vi "ScopeIntegrateSignal_v3.vi"() -> ()   [LabVIEW 2018]
doc: "This example illustrates how to use autosetup and continuously acquires waveforms from a single channel using the following steps:\n\n1. Specify a valid VISA session. \n2. Specify a channel. \n3. Specify a time-out value for reading waveform.\n4. Run the VI. The graph displays the waveform you acquire."
uses:
  <vilib>/Analysis/baseanly.llb/Mean (DBL).vi
  <instrlib>/Tektronix DPO MSO 2000 4000 Series/Public/Data/Read (Single Waveform).vi
  <vilib>/Waveform/WDTFileIO.llb/Export Waveform To Spreadsheet File.vi
  <instrlib>/Tektronix DPO MSO 2000 4000 Series/Tektronix DPO MSO 2000 4000 Series.lvlib
  <vilib>/Analysis/NI_AALBase.lvlib
panel:
  in  "Save waveform?":bool
  in  "autocurs":bool=TRUE
  out "roi_stop":i64=496919
  out "roi_start":i64=496793
  in  "thresh":dbl=0.30000000000000004 format="%#_13g"
  in  "acquire":bool=TRUE
  in  "milliseconds to wait":u32=100
  out "Numeric":i32
  out "standard deviation":dbl=-0.0 format="%0.2f"
  out "mean":dbl=nan format="%0.2f"
  in  "Looping?":bool
  in  "stop":bool
  out "integrated signal array":dbl[](array[numeric])=[5.081550747205201e-09]
  out "bkgd":dbl=-0.0005882788252936317 format="%0.5f"
  out "bkgd stop":dbl=0.00019852
  out "bkgd start":dbl=5.636363636363637e-05
  out "dt":dbl=4e-10
  out "integral (nVs)":sgl=5.0815506
  out "stop int":dbl=0.00019876854
  out "start int":dbl=0.00019871893000000001
  in  "Channel (0: Channel 1)":u16(ring)=2 items=["Channel 1", "Channel 2", "Channel 3", "Channel 4", "Math", "Reference 1", "Reference 2", "Reference 3", "Reference 4"]
  in  "Maximum Time (10000ms)":u32=10000
  in  "VISA Resource Name":refnum<visa-resource-name>="mdo4034c"
  out "Waveform Graph":waveform(dbl)(graph)={"t0"=timestamp(-0.0001988000000000545 s since 1904-01-01), "dt"=4e-10, "Y"=array[1000000 elements]}
  # "(C) 2006 - 2022. National Instruments Corporation. ALL RIGHTS RESERVED."
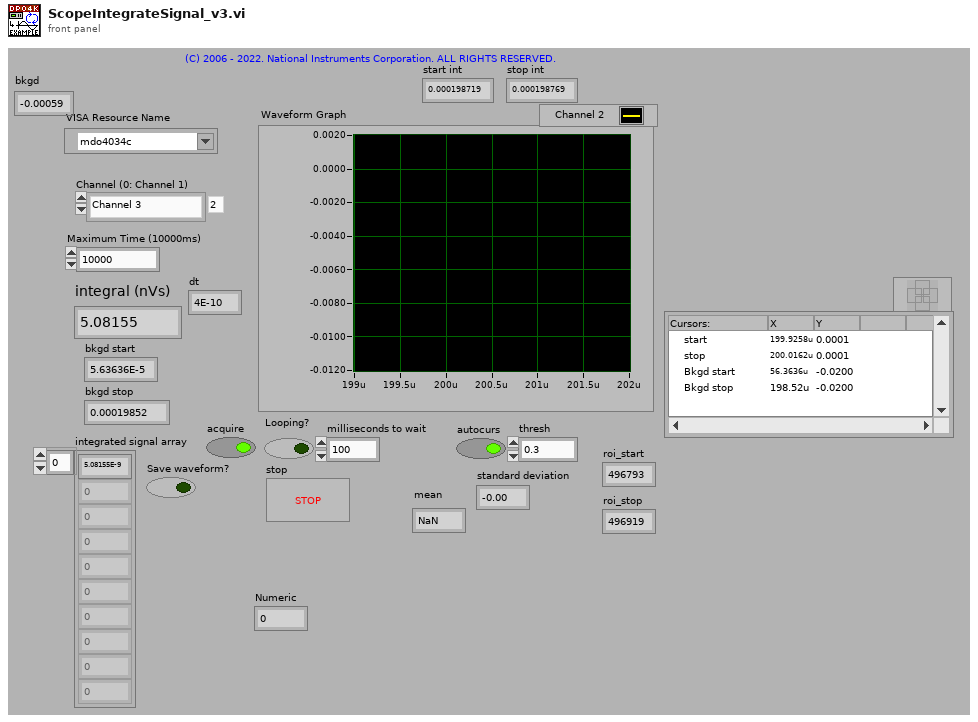
[diagram p1: front panel]
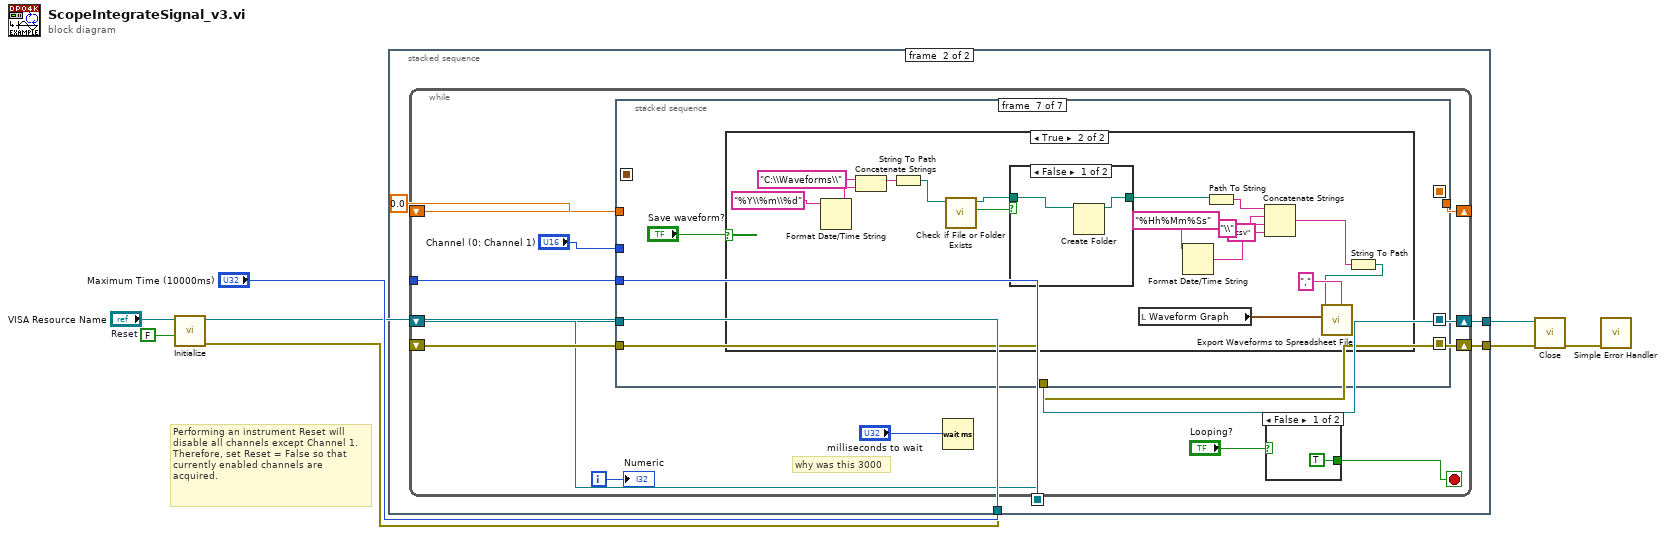
[diagram p0: block diagram]
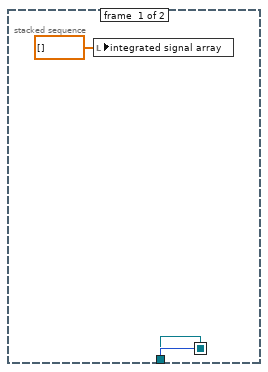
[diagram p2: hidden frame]
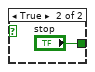
[diagram p3: hidden frame]
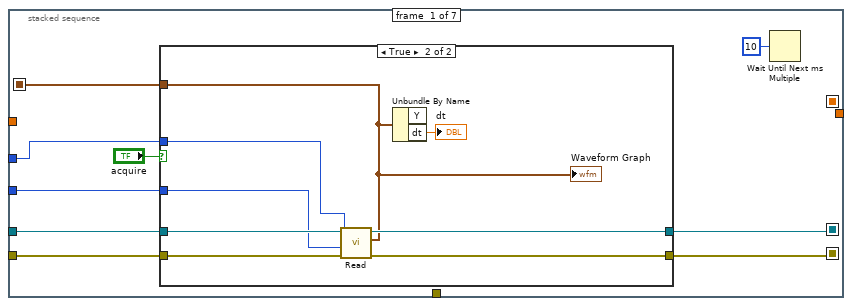
[diagram p4: hidden frame]
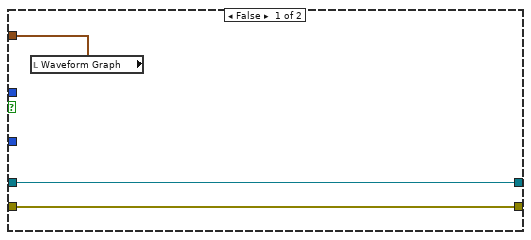
[diagram p5: hidden frame]
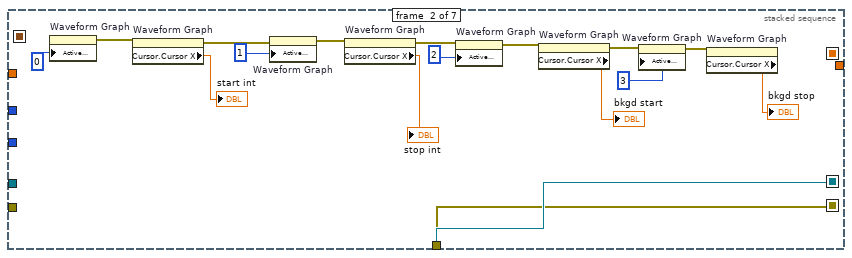
[diagram p6: hidden frame]
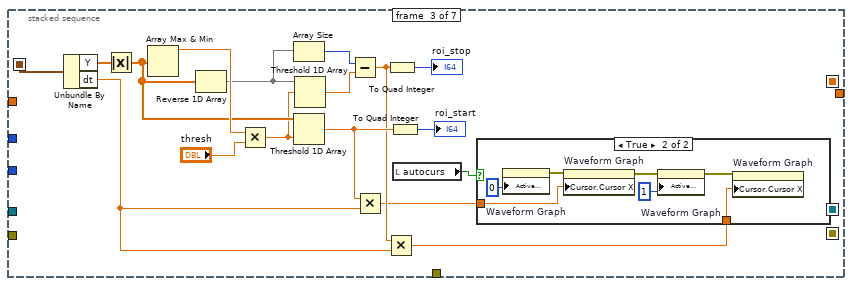
[diagram p7: hidden frame]
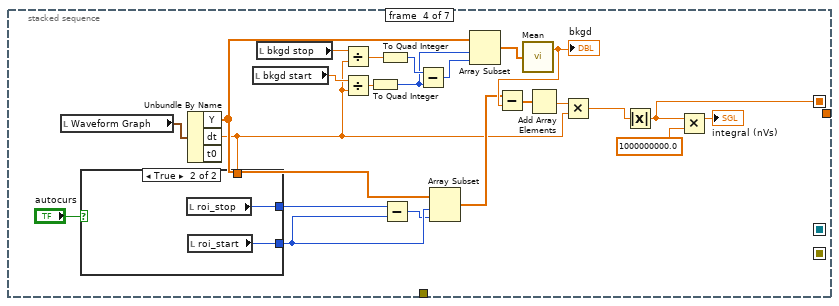
[diagram p9: hidden frame]
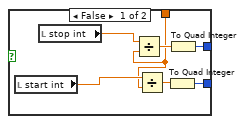
[diagram p10: hidden frame]
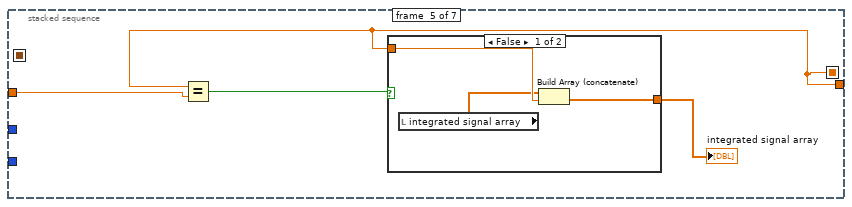
[diagram p11: hidden frame]
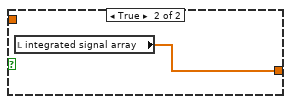
[diagram p12: hidden frame]
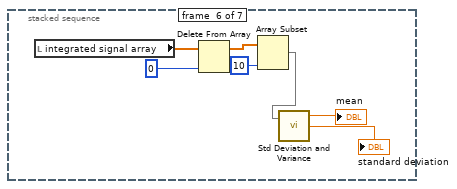
[diagram p13: hidden frame]
diagram:
  w4 = FALSE  # Reset
  # "Performing an instrument Reset will disable all channels except Channel 1. Therefore, set Reset = False so that currently enabled channels are acquired."
  n1 = call <instrlib>:"Initialize.vi"("Reset (True)"=w4, "VISA resource name"="VISA Resource Name") -> ("error out"=w2:errorcluster, "VISA resource name out"=w1:refnum<visa-resource-name>)  [unwired: 8 in]
  n2 = stacked-sequence {
    seq-local: [w12 _] -> [_ w16]
    seq-local: [w11 _] -> [_ w15]
    seq-local: [w10 _] -> [_ w14]
    tunnel: "Maximum Time (10000ms)" -> [w12 _]
    tunnel: w2 -> [w11 _]
    tunnel: w1 -> [w10 _]
    tunnel: [_ w18] -> w7
    tunnel: [_ w17] -> w6
    frame #0 {
      n3 = local write "integrated signal array"(dbl[] [] ("integrated signal array")) -> ()
    }
    frame #1 {
      n4 = while {
        tunnel: w16 -> [w28]
        shift-right: [w29] -> w17
        shift-left: w15 -> [w27]
        shift-right: [w30] -> w18
        shift-left: w14 -> [w26]
        shift-right: [w25] -> _
        shift-left: 0.0 -> [w24]
        i -> [w21]
        stop <- w22 stop-if-true
        # "why was this 3000"
        n5 = stacked-sequence {
          seq-local: [w39 _ _ _ _ _ _] -> [_ w69 _ _ _ _ _]
          seq-local: [w37 _ _ _ _ _ _] -> [_ w68 _ _ _ _ _]
          seq-local: [_ _ _ w101 _ _ _] -> [_ _ _ _ w127 _ _]
          seq-local: [w33 _ _ _ _ _ _] -> [_ _ w86 _ _ _ _]
          tunnel: w26 -> [w41 _ _ _ _ _ _]
          tunnel: w27 -> [w40 _ _ _ _ _ _]
          tunnel: w28 -> [w36 _ _ _ _ _ _]
          tunnel: "Channel (0: Channel 1)" -> [w35 _ _ _ _ _ _]
          tunnel: [_ w69 _ _ _ _ _] -> w30
          tunnel: [_ w68 _ _ _ _ _] -> w29
          tunnel: [_ _ _ _ w127 _ _] -> w25
          tunnel: w24 -> [_ _ _ _ w126 _ _]
          frame #0 {
            n6 = case shown="True" "acquire" {
              tunnel: w41 -> [w44 w52]
              tunnel: w40 -> [w43 w51]
              tunnel: [w44 w50] -> w39
              tunnel: [w43 w49] -> w37
              tunnel: w36 -> [_ w48]
              tunnel: w35 -> [_ w46]
              tunnel: [w42 w45] -> w33
              frame False {
                n7 = local read "Waveform Graph"() -> (w42:waveform(dbl))
              }
              frame True {
                n8 = call-poly <instrlib>:"Read.vi"("error in (no error)"=w51, "Maximum Time (10000ms)"=w48, "Channel (0: Channel 1)"=w46, "VISA resource name"=w52) -> ("error out"=w49:errorcluster, "Waveform Graph"=w45:waveform(dbl), "VISA resource name out"=w50:refnum<visa-resource-name>)  [unwired: 5 in]
                "Waveform Graph" <- w45
                n9 = Unbundle By Name(w45) -> ("dt"=→"dt":dbl)  [unwired: 1 out]
              }
            }
            n10 = Wait Until Next ms Multiple(millisecond multiple=u32 10) -> ()  [unwired: 1 out]
          }
          frame #1 {
            n11 = property on="Waveform Graph" class="WFGraph (strict)"("Active Cursor"=0 ("Cursor.Cursor Index")) -> (error out=w66:errorcluster)  [unwired: 2 in, 1 out]
            n12 = property on="Waveform Graph" class="WFGraph (strict)"(error in=w66) -> (error out=w65:errorcluster, "Cursor.Cursor X"=→"start int":dbl)  [unwired: 1 in, 1 out]
            n13 = property on="Waveform Graph" class="WFGraph (strict)"(error in=w65, "Active Cursor"=1 ("Cursor.Cursor Index")) -> (error out=w64:errorcluster)  [unwired: 1 in, 1 out]
            n14 = property on="Waveform Graph" class="WFGraph (strict)"(error in=w64) -> (error out=w59:errorcluster, "Cursor.Cursor X"=→"stop int":dbl)  [unwired: 1 in, 1 out]
            n15 = property on="Waveform Graph" class="WFGraph (strict)"(error in=w59, "Active Cursor"=u32 2) -> (error out=w60:errorcluster)  [unwired: 1 in, 1 out]
            n16 = property on="Waveform Graph" class="WFGraph (strict)"(error in=w60) -> (error out=w56:errorcluster, "Cursor.Cursor X"=→"bkgd start":dbl)  [unwired: 1 in, 1 out]
            n17 = property on="Waveform Graph" class="WFGraph (strict)"(error in=w56, "Active Cursor"=u32 3) -> (error out=w57:errorcluster)  [unwired: 1 in, 1 out]
            n18 = property on="Waveform Graph" class="WFGraph (strict)"(error in=w57) -> ("Cursor.Cursor X"=→"bkgd stop":dbl)  [unwired: 1 in, 2 out]
          }
          frame #2 {
            n19 = Unbundle By Name(w86) -> ("Y"=w85:dbl[], "dt"=w73:dbl)
            n20 = Absolute Value(x=w85) -> (abs(x)=w82:dbl[])
            n21 = Array Max & Min(array=w82) -> (max value=w84:dbl)  [unwired: 3 out]
            n22 = Reverse 1D Array(array=w82) -> (reversed array=w80:dbl[])
            n23 = Multiply(x=w84, y="thresh") -> (x*y=w81:dbl)
            n24 = Array Size(array=w80) -> (size(s)=w79:i32)
            n25 = Threshold 1D Array(2:w81, 3:w82) -> (0:w75:dbl)  [unwired: 1 in]
            n26 = Threshold 1D Array(2:w81, 3:w80) -> (0:w78:dbl)  [unwired: 1 in]
            n27 = Subtract(x=w79, y=w78) -> (x-y=w74:dbl)
            n28 = Multiply(x=w75, y=w73) -> (x*y=w71:dbl)
            n29 = Multiply(x=w74, y=w73) -> (x*y=w72:dbl)
            n30 = To Quad Integer(1:w74) -> (0:→"roi_stop":i64)
            n31 = To Quad Integer(1:w75) -> (0:→"roi_start":i64)
            n32 = local read "autocurs"() -> (w70:bool)
            n33 = case shown="True" w70 {
              tunnel: w72 -> [_ w88]
              tunnel: w71 -> [_ w87]
              frame False {
              }
              frame True {
                n34 = property on="Waveform Graph" class="WFGraph (strict)"("Active Cursor"=0 ("Cursor.Cursor Index")) -> (error out=w93:errorcluster)  [unwired: 2 in, 1 out]
                n35 = property on="Waveform Graph" class="WFGraph (strict)"(error in=w93, "Cursor.Cursor X"=w87) -> (error out=w92:errorcluster)  [unwired: 1 in, 1 out]
                n36 = property on="Waveform Graph" class="WFGraph (strict)"(error in=w92, "Active Cursor"=1 ("Cursor.Cursor Index")) -> (error out=w91:errorcluster)  [unwired: 1 in, 1 out]
                n37 = property on="Waveform Graph" class="WFGraph (strict)"(error in=w91, "Cursor.Cursor X"=w88) -> ()  [unwired: 1 in, 2 out]
              }
            }
          }
          frame #3 {
            n38 = local read "Waveform Graph"() -> (w113:waveform(dbl))
            n39 = Unbundle By Name(w113) -> ("Y"=w112:dbl[], "dt"=w96:dbl)  [unwired: 1 out]
            n40 = case shown="True" "autocurs" {
              tunnel: [w119 w124] -> w116
              tunnel: [w118 w125] -> w115
              tunnel: w96 -> [w117 _]
              frame False {
                n41 = local read "start int"() -> (w122:dbl)
                n42 = local read "stop int"() -> (w123:dbl)
                n43 = Divide(x=w123, y=w117) -> (x/y=w121:dbl)
                n44 = Divide(x=w122, y=w117) -> (x/y=w120:dbl)
                n45 = To Quad Integer(1:w120) -> (0:w118:i64)
                n46 = To Quad Integer(1:w121) -> (0:w119:i64)
              }
              frame True {
                n47 = local read "roi_stop"() -> (w124:i64)
                n48 = local read "roi_start"() -> (w125:i64)
              }
            }
            n49 = local read "bkgd start"() -> (w108:dbl)
            n50 = local read "bkgd stop"() -> (w109:dbl)
            n51 = Divide(x=w109, y=w96) -> (x/y=w110:dbl)
            n52 = Divide(x=w108, y=w96) -> (x/y=w111:dbl)
            n53 = To Quad Integer(1:w111) -> (0:w105:i64)
            n54 = To Quad Integer(1:w110) -> (0:w107:i64)
            n55 = Subtract(x=w116, y=w115) -> (x-y=w114:i64)
            n56 = Subtract(x=w107, y=w105) -> (x-y=w106:i64)
            n57 = Array Subset(array=w112, index=w115, length=w114) -> (w102:dbl[])
            n58 = Array Subset(array=w112, index=w105, length=w106) -> (w104:dbl[])
            n59 = call-poly <vilib>:"Mean.vi"("X"=w104) -> ("mean"=w103:dbl)  [unwired: 1 out]
            "bkgd" <- w103
            n60 = Subtract(x=w102, y=w103) -> (x-y=w98:dbl[])
            n61 = Add Array Elements(numeric array=w98) -> (sum=w97:dbl)
            n62 = Multiply(x=w97, y=w96) -> (x*y=w95:dbl)
            n63 = Absolute Value(x=w95) -> (abs(x)=w101:dbl)
            n64 = Multiply(x=w101, y=1000000000.0) -> (x*y=→"integral (nVs)":dbl)
          }
          frame #4 {
            n65 = Equal?(x=w127, y=w126) -> (x = y?=w129:bool)
            n66 = case shown="False" w129 {
              tunnel: w127 -> [w132 _]
              tunnel: [w131 w133] -> w128
              frame False {
                n67 = local read "integrated signal array"() -> (w130:dbl[])
                n68 = Build Array (concatenate)(w130, w132) -> (w131:dbl[])
              }
              frame True {
                n69 = local read "integrated signal array"() -> (w133:dbl[])
              }
            }
            "integrated signal array" <- w128
          }
          frame #5 {
            n70 = local read "integrated signal array"() -> (w140:dbl[])
            n71 = Delete From Array(array=w140, index=0) -> (array with subset deleted=w136:dbl[])  [unwired: 1 in, 1 out]
            n72 = Array Subset(array=w136, length=10) -> (w135:dbl[])  [unwired: 1 in]
            n73 = call <vilib>:"Std Deviation and Variance.vi"("X"=w135) -> ("mean"=→"mean":dbl, "standard deviation"=→"standard deviation":dbl)  [unwired: 1 in, 1 out]
          }
          frame #6 {
            n74 = case shown="True" "Save waveform?" {
              frame False {
              }
              frame True {
                n75 = Format Date/Time String(time format string (%c)="%Y\\%m\\%d") -> (date/time string=w155:string)  [unwired: 2 in]
                n76 = Concatenate Strings("C:\\Waveforms\\" ("string"), w155) -> (w156:string)
                n77 = String To Path(string=w156) -> (path=w153:path)
                n78 = call <vilib>:"Check if File or Folder Exists.vi"("path"=w153) -> ("file or folder exists?"=w151:bool, "dup path"=w150:path)  [unwired: 8 in, 1 out]
                n79 = case shown="False" w151 {
                  tunnel: w150 -> [w160 w161]
                  tunnel: [w159 w161] -> w149
                  frame False {
                    n80 = Create Folder(path (use dialog)=w160) -> (created path=w159:path)  [unwired: 2 in, 2 out]
                  }
                  frame True {
                  }
                }
                n81 = local read "Waveform Graph"() -> (w158:waveform(dbl))
                n82 = Format Date/Time String(time format string (%c)="%Hh%Mm%Ss") -> (date/time string=w145:string)  [unwired: 2 in]
                n83 = Path To String(path=w149) -> (string=w148:string)
                n84 = Concatenate Strings(w148, "\\" ("string"), w145, ".csv" ("string")) -> (w144:string)
                n85 = String To Path(string=w144) -> (path=w143:path)
                n86 = call-poly <vilib>:"Export Waveforms to Spreadsheet File.vi"("delimiter (Tab)"=",", "waveform"=w158, "file path (dialog if empty)"=w143) -> ()  [unwired: 7 in, 2 out]
              }
            }
          }
        }
        n87 = Wait (ms)(milliseconds to wait="milliseconds to wait") -> ()  [unwired: 1 out]
        n88 = case shown="False" "Looping?" {
          tunnel: [TRUE ("stop") "stop"] -> w22
          frame False {
          }
          frame True {
          }
        }
        "Numeric" <- w21
      }
    }
  }
  n89 = call <instrlib>:"Close.vi"("error in (no error)"=w6, "VISA resource name"=w7) -> ("error out"=w5:errorcluster)  [unwired: 9 in]
  n90 = call <vilib>:"Simple Error Handler.vi"("error in (no error)"=w5) -> ()  [unwired: 4 in, 5 out]
